vi "Page_Source_Can_Add_To_Bottom.vi"(8 "error in (no error)":errorcluster, 11 "AB_Source_VI in":refnum<class "AB_Source_VI.lvclass">) -> (0 "error out":errorcluster, 1 "message":string, 2 "canAddToBottom":bool, 3 "AB_Source_VI out":refnum<class "AB_Source_VI.lvclass">)   [LabVIEW 2020, in "AB_Source_VI.lvclass"]
uses:
  <vilib>/AppBuilder/AB_Classes/Source/VI/AB_Source_VI.lvclass
  <vilib>/AppBuilder/AB_Classes/Source/VI/AB_Source_VI.lvclass/AB_Source_VI.ctl
  <resource>/Framework/Providers/Common/provcom_StringGlobals.vi
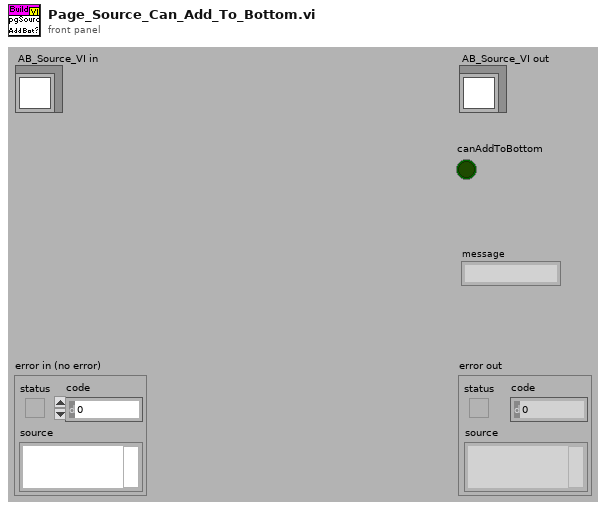
[diagram p1: front panel]
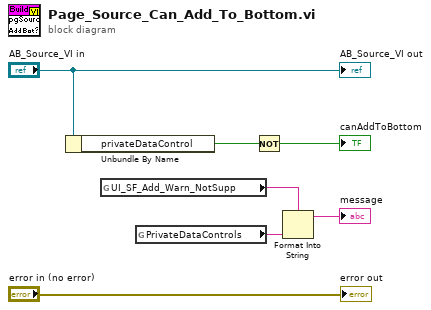
[diagram p0: block diagram]
diagram:
  n1 = Unbundle By Name("AB_Source_VI in") -> ("privateDataControl"=w5:bool)
  n2 = global read "provcom_StringGlobals.vi" "UI_SF_Add_Warn_NotSupp"() -> (w3:string)
  n3 = global read "provcom_StringGlobals.vi" "PrivateDataControls"() -> (w1:string)
  n4 = Not(x=w5) -> (.not. x?=→"canAddToBottom":bool)
  n5 = Format Into String(format string=w3, w1) -> (resulting string=→"message":string)  [unwired: 2 in, 1 out]
  "error out" <- "error in (no error)"
  "AB_Source_VI out" <- "AB_Source_VI in"
